vi "Set all f same.vi"(8 "error in (no error)":errorcluster, 11 "Instrument.DAQ":refnum<class "Instrument.DAQ.lvclass">) -> (0 "error out":errorcluster, 3 "Instrument.DAQ out":refnum<class "Instrument.DAQ.lvclass">)   [LabVIEW 2019, in "Instrument.Lockin.lvlib" / "Instrument.DAQ.lvclass"]
uses:
  Instrument.DAQ.lvclass
  Instrument.DAQ.lvclass/Instrument.DAQ.ctl
panel:
  # "4"
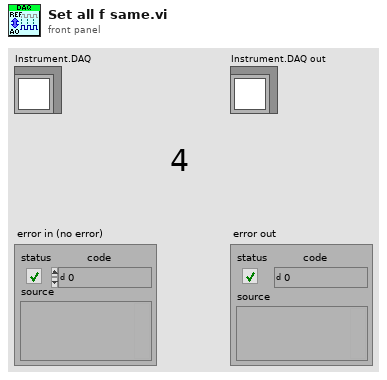
[diagram p1: front panel]
types:
  T1 = typedef "Instrument.Lockin.lvlib/Instrument.DAQ.lvclass/AO.Channel--Cluster--Array.ctl" = T2[]
  T2 = typedef "Instrument.Lockin.lvlib/Instrument.DAQ.lvclass/AO.Channel--Cluster.ctl" = cluster{"Enable?":bool, "Channel":i32, "Amplitude":dbl, "Offset":dbl, "Frequency":dbl, "Phase":dbl, "Function":T3, "Sweeping?":bool, "Limit AC":bool, "Limit DC?":bool, "Duty Cycle":bool}
  T3 = typedef "Instrument.Lockin.lvlib/Instrument.DAQ.lvclass/AO.Channel.Function--Enum.ctl" = enum16{"sine", "square", "triangle", "saw"}
  T4 = typedef "Instrument.Lockin.lvlib/Instrument.DAQ.lvclass/REF.Channel--Cluster--Array.ctl" = T5[]
  T5 = typedef "Instrument.Lockin.lvlib/Instrument.DAQ.lvclass/REF.Channel--Cluster.ctl" = cluster{"Enable?":bool, "Channel":i32, "Frequency":dbl, "Phase":dbl, "TC":dbl, "Roll-Off":i32}
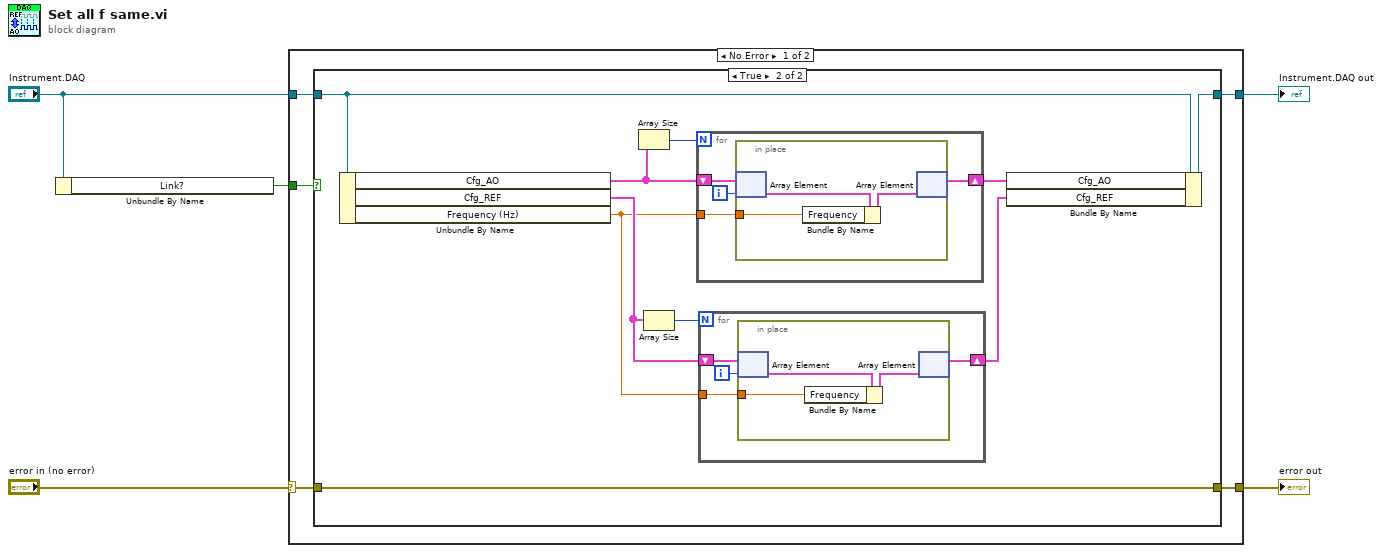
[diagram p0: block diagram]
diagram:
  n1 = Unbundle By Name("Instrument.DAQ") -> ("Link?"=w2:bool)
  n2 = case shown="No Error" "error in (no error)" {
    selector: "error in (no error)" -> [w8 w38]
    tunnel: "Instrument.DAQ" -> [w10 w37]
    tunnel: [w9 w37] -> w1
    tunnel: [w7 w38] -> w4
    tunnel: w2 -> [w6 _]
    frame No Error {
      n3 = case shown="True" w6 {
        tunnel: w10 -> [w11 w22]
        tunnel: [w11 w21] -> w9
        tunnel: w8 -> [w12 w19]
        tunnel: [w12 w19] -> w7
        frame False {
        }
        frame True {
          n4 = Unbundle By Name(w22) -> ("Cfg_AO"=w18:T1, "Cfg_REF"=w15:T4, "Frequency (Hz)"=w14:dbl)
          n5 = Array Size(array=w18) -> (size(s)=w17:i32)
          n6 = Array Size(array=w15) -> (size(s)=w16:i32)
          n7 = for {
            N: w17 -> [_]
            tunnel: w14 -> [w26]
            shift-right: [w23] -> w20
            shift-left: w18 -> [w25]
            i -> [w24]
            n8 = in-place {
              in-place-border: w26 -> [w29]
              n9 = in-place-array #1(w25, w24) -> (w28:T2)
              n10 = Bundle By Name(cluster=w28, "Frequency"=w29) -> (w27:T2)
              n11 = in-place-array #1(w27) -> (w23:T1)  [unwired: 1 out]
            }
          }
          n12 = for {
            N: w16 -> [_]
            tunnel: w14 -> [w33]
            shift-right: [w30] -> w13
            shift-left: w15 -> [w32]
            i -> [w31]
            n13 = in-place {
              in-place-border: w33 -> [w36]
              n14 = in-place-array #2(w32, w31) -> (w35:T5)
              n15 = Bundle By Name(cluster=w35, "Frequency"=w36) -> (w34:T5)
              n16 = in-place-array #2(w34) -> (w30:T4)  [unwired: 1 out]
            }
          }
          n17 = Bundle By Name(cluster=w22, "Cfg_AO"=w20, "Cfg_REF"=w13) -> (w21:refnum<class "Instrument.DAQ.lvclass">)
        }
      }
    }
    frame Error {
    }
  }
  "error out" <- w4
  "Instrument.DAQ out" <- w1
